vi "Write DO.vi"(0 "FPGA DO Loop Data in":T1={"DO"=[FALSE, FALSE, FALSE, FALSE, FALSE, FALSE, FALSE, FALSE, FALSE, FALSE, FALSE, FALSE, FALSE, FALSE, FALSE, FALSE, FALSE, FALSE, FALSE, FALSE, FALSE, FALSE, FALSE, FALSE, FALSE, FALSE, FALSE, FALSE, FALSE, FALSE, FALSE, FALSE], "Is Pulse"=[FALSE, FALSE, FALSE, FALSE, FALSE, FALSE, FALSE, FALSE, FALSE, FALSE, FALSE, FALSE, FALSE, FALSE, FALSE, FALSE, FALSE, FALSE, FALSE, FALSE, FALSE, FALSE, FALSE, FALSE, FALSE, FALSE, FALSE, FALSE, FALSE, FALSE, FALSE, FALSE], "Set Time uSec"=[0, 0, 0, 0, 0, 0, 0, 0, 0, 0, 0, 0, 0, 0, 0, 0, 0, 0, 0, 0, 0, 0, 0, 0, 0, 0, 0, 0, 0, 0, 0, 0], "Wait Time uSec"=[0, 0, 0, 0, 0, 0, 0, 0, 0, 0, 0, 0, 0, 0, 0, 0, 0, 0, 0, 0, 0, 0, 0, 0, 0, 0, 0, 0, 0, 0, 0, 0]}) -> (4 "FPGA DO Loop Data out":T1, 6 "DO":u32, 15 "error out":errorcluster)   [LabVIEW 2019]
uses:
  TypeDef/FPGA DO Loop Data.ctl
  <vilib>/rvi/Emulation/niFpgaEmulationIsFPGAContextNoSignature.vi
  <vilib>/rvi/Emulation/niFpgaSctlEmulationGetInTimedLoop.vi
  <vilib>/rvi/errors/niFpgaSetErrorForExecOnDevCompSimple.vi
  <vilib>/rvi/eio/common/nirviEmuReportErrorAndStop.vi
  <vilib>/rvi/DataTransferAndStorage/Container/Common/niFpgaContainerGetUniqueNameForEmu.vi
  <vilib>/rvi/FIFO/Fifo_Resource/nirvififoEmulationSetSize.vi
  <vilib>/rvi/FIFO/Fifo_Resource/nirviFifoEmulationQueueMgr.vi
  <instcachedir>/0/nirviFifoEmulationQueueMgr_E5CAEC123FF24DC58D834DCA3CDAA9B5.lvgen/nirviFifoEmulationQueueMgr_E5CAEC123FF24DC58D834DCA3CDAA9B5_002.vi
  <vilib>/Utility/error.llb/Clear Errors.vi
  <vilib>/rvi/FIFO/Fifo_Resource/nirvififoEmulationCreateLock.vi
  <vilib>/rvi/Emulation/niFpgaProcessEmulError.vi
  <vilib>/rvi/FIFO/Fifo_Resource/nirvififoEmulationObtainLock.vi
  <vilib>/rvi/FIFO/Fifo_Resource/nirvififoEmulationReleaseLock.vi
  <vilib>/rvi/occurrence/nirviWaitOnOccurrenceBase.vi
  <vilib>/rvi/errors/nirviReportUnexpectedCaseInternalError.vi
  <vilib>/rvi/errors/nirviReportUnexpectedCaseInternalError (U32).vi
  <vilib>/rvi/eio/common/nirviEmuTemplateMethod_errors.vi
  <vilib>/rvi/DataTransferAndStorage/Container/XNode/niFpgaContainer.xnode
  <vilib>/rvi/FIFO/Fifo_Resource/nirvififoEmulationRead.vi
  <vilib>/eio/EIONode/EIONode.xnode
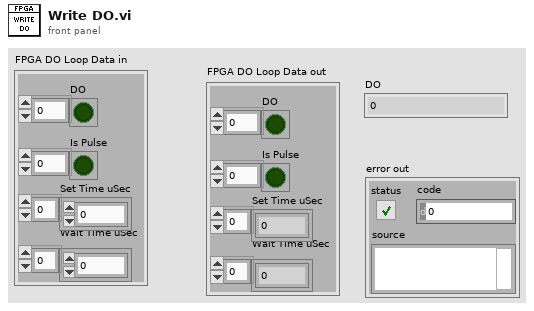
[diagram p1: front panel]
types:
  T1 = typedef "FPGA DO Loop Data.ctl" = cluster{"DO":bool[], "Is Pulse":bool[], "Set Time uSec":u32[], "Wait Time uSec":u32[]}
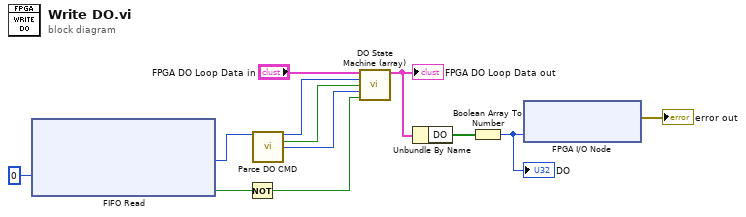
[diagram p0: block diagram]
diagram:
  n1 = xnode "FIFO Read"("Timeout"=0) -> ("Element"=w2:u64, "Timed Out?"=w1:bool)  [unwired: 1 in, 1 out]
  n2 = Not(x=w1) -> (.not. x?=w11:bool)
  n3 = call "Parce DO CMD.vi"("CMD"=w2) -> ("#DO"=w10:u8, "Value"=w9:bool, "Time uSec"=w8:u32)  [unwired: 12 in]
  n4 = call "DO State Machine (array).vi"("FPGA DO Loop Data in"="FPGA DO Loop Data in", "#DO"=w10, "Value"=w9, "Time uSec"=w8, "Set"=w11) -> ("FPGA DO Loop Data out"=w6:T1)  [unwired: 10 in]
  "FPGA DO Loop Data out" <- w6
  n5 = Unbundle By Name(w6) -> ("DO"=w5:bool[])
  n6 = Boolean Array To Number(Boolean array=w5) -> (number=w4:u32)
  "DO" <- w4
  n7 = xnode "FPGA I/O Node"("Mod2/DO31:0"=w4) -> ("error out"=→"error out":errorcluster)  [unwired: 2 in, 1 out]
